vi "CCD Target.vi"(8 "error in (no error)":errorcluster, 11 "Image":T1) -> (0 "error out":errorcluster={"status"=TRUE, "code"=-1074396120, "source"="IMAQ Clear Image Overlay\n  "}, 3 "Image Out":T1)   [LabVIEW 2015, in "CCD.lvlib"]
uses:
  CCD.lvlib
  <vilib>/vision/Image Controls.llb/IMAQ Image.ctl
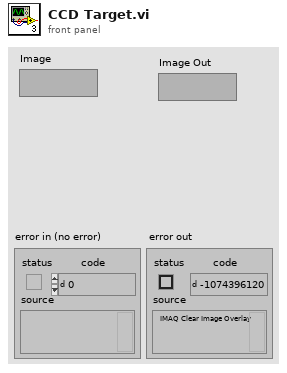
[diagram p1: front panel]
types:
  T1 = typedef "IMAQ Image.ctl" = refnum<image>
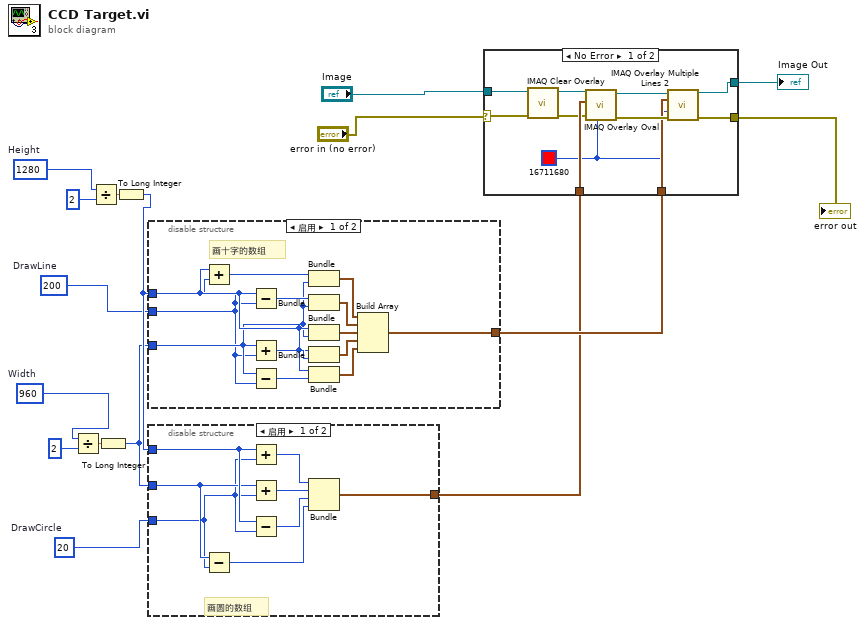
[diagram p0: block diagram]
diagram:
  w2 = 20  # DrawCircle
  w5 = 960  # Width
  w3 = 200  # DrawLine
  w11 = 1280  # Height
  n1 = Divide(x=w5, y=2) -> (x/y=w6:dbl)
  n2 = Divide(x=w11, y=2) -> (x/y=w8:dbl)
  n3 = To Long Integer(number=w6) -> (32bit integer=w4:i32)
  n4 = To Long Integer(number=w8) -> (32bit integer=w9:i32)
  n5 = disable-structure shown="启用" {
    disable-tunnel: w9 -> [w20 _]
    disable-tunnel: w4 -> [w19 _]
    disable-tunnel: [w18 _] -> w16
    disable-tunnel: w3 -> [w17 _]
    frame Enabled {
      # "画十字的数组"
      n6 = Add(x=w20, y=w17) -> (x+y=w29:i32)
      n7 = Subtract(x=w20, y=w17) -> (x-y=w28:i32)
      n8 = Add(x=w19, y=w17) -> (x+y=w27:i32)
      n9 = Subtract(x=w19, y=w17) -> (x-y=w26:i32)
      n10 = Bundle(w29, w19) -> (w25:cluster{i32, i32})  [unwired: 1 in]
      n11 = Bundle(w28, w19) -> (w24:cluster{i32, i32})  [unwired: 1 in]
      n12 = Bundle(w20, w19) -> (w23:cluster{i32, i32})  [unwired: 1 in]
      n13 = Bundle(w20, w27) -> (w22:cluster{i32, i32})  [unwired: 1 in]
      n14 = Bundle(w20, w26) -> (w21:cluster{i32, i32})  [unwired: 1 in]
      n15 = Build Array(w25, w24, w23, w22, w21) -> (w18:cluster{i32, i32}[])
    }
    frame Disabled {
    }
  }
  n16 = disable-structure shown="启用" {
    disable-tunnel: w9 -> [w33 _]
    disable-tunnel: w4 -> [w32 _]
    disable-tunnel: [w31 _] -> w15
    disable-tunnel: w2 -> [w30 _]
    frame Enabled {
      # "画圆的数组"
      n17 = Subtract(x=w32, y=w30) -> (x-y=w36:i32)
      n18 = Add(x=w33, y=w30) -> (x+y=w37:i32)
      n19 = Add(x=w32, y=w30) -> (x+y=w35:i32)
      n20 = Subtract(x=w33, y=w30) -> (x-y=w34:i32)
      n21 = Bundle(w37, w35, w34, w36) -> (w31:cluster{i32, i32, i32, i32})  [unwired: 1 in]
    }
    frame Disabled {
    }
  }
  n22 = case shown="No Error" "error in (no error)" {
    selector: "error in (no error)" -> [w38 w49]
    tunnel: w16 -> [w46 _]
    tunnel: w15 -> [w45 _]
    tunnel: [w43 w50] -> w14
    tunnel: [w42 w49] -> w13
    tunnel: "Image" -> [w39 w50]
    frame No Error {
      w44 = u32 16711680 ("Color")
      n23 = call "IMAQ Clear Overlay"("error in (no error)"=w38, "Image"=w39) -> ("error out"=w40:errorcluster, "Image Out"=w41:T1)  [unwired: 8 in]
      n24 = call "IMAQ Overlay Oval"("Color"=w44, "error in (no error)"=w40, "Bounding Rectangle"=w45, "Image"=w41) -> ("error out"=w48:errorcluster, "Image Out"=w47:T1)  [unwired: 6 in]
      n25 = call "IMAQ Overlay Multiple Lines 2"("Image"=w47, "Line End Points"=w46, "Color"=w44, "error in (no error)"=w48) -> ("Image Out"=w43:T1, "error out"=w42:errorcluster)  [unwired: 10 in]
    }
    frame Error {
    }
  }
  "Image Out" <- w14
  "error out" <- w13
